vi "Update Function Variables.vi"(8 "error in (no error)":errorcluster, 10 "Variable Names":string[](array[string]), 11 "Structure Loop in":refnum<class "functionbase.lvclass">) -> (0 "error out":errorcluster, 3 "Structure Loop out":refnum<class "functionbase.lvclass">)   [LabVIEW 2019, in "LSL.lvlib" / "functionbase.lvclass"]
uses:
  functionbase.lvclass
  functionbase.lvclass/functionbase.ctl
  properties/Read Func Full String.vi
  properties/Read RT Variables.vi
  variables/RT Variables/RT Variables.lvclass
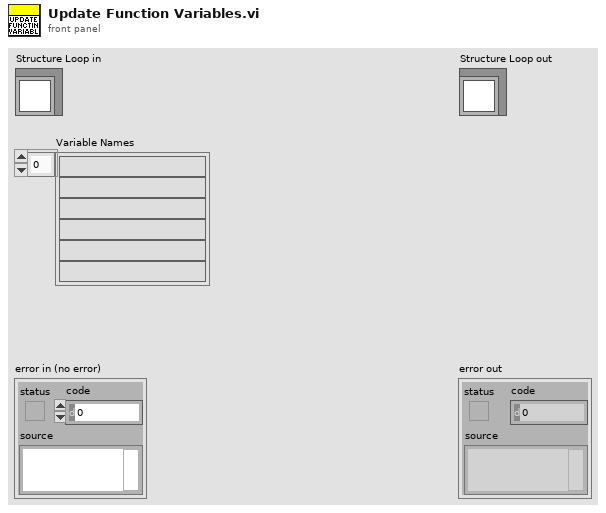
[diagram p1: front panel]
types:
  T1 = typedef "Datatype.ctl" = enum16{"Null", "Numeric", "String", "Bool", "Numeric 1D", "String 1D", "Bool 1D", "Numeric 2D", "String 2D", "Bool 2D", "Variant"}
  T2 = typedef "Valuetype.ctl" = enum16{"Value", "Variable", "Function"}
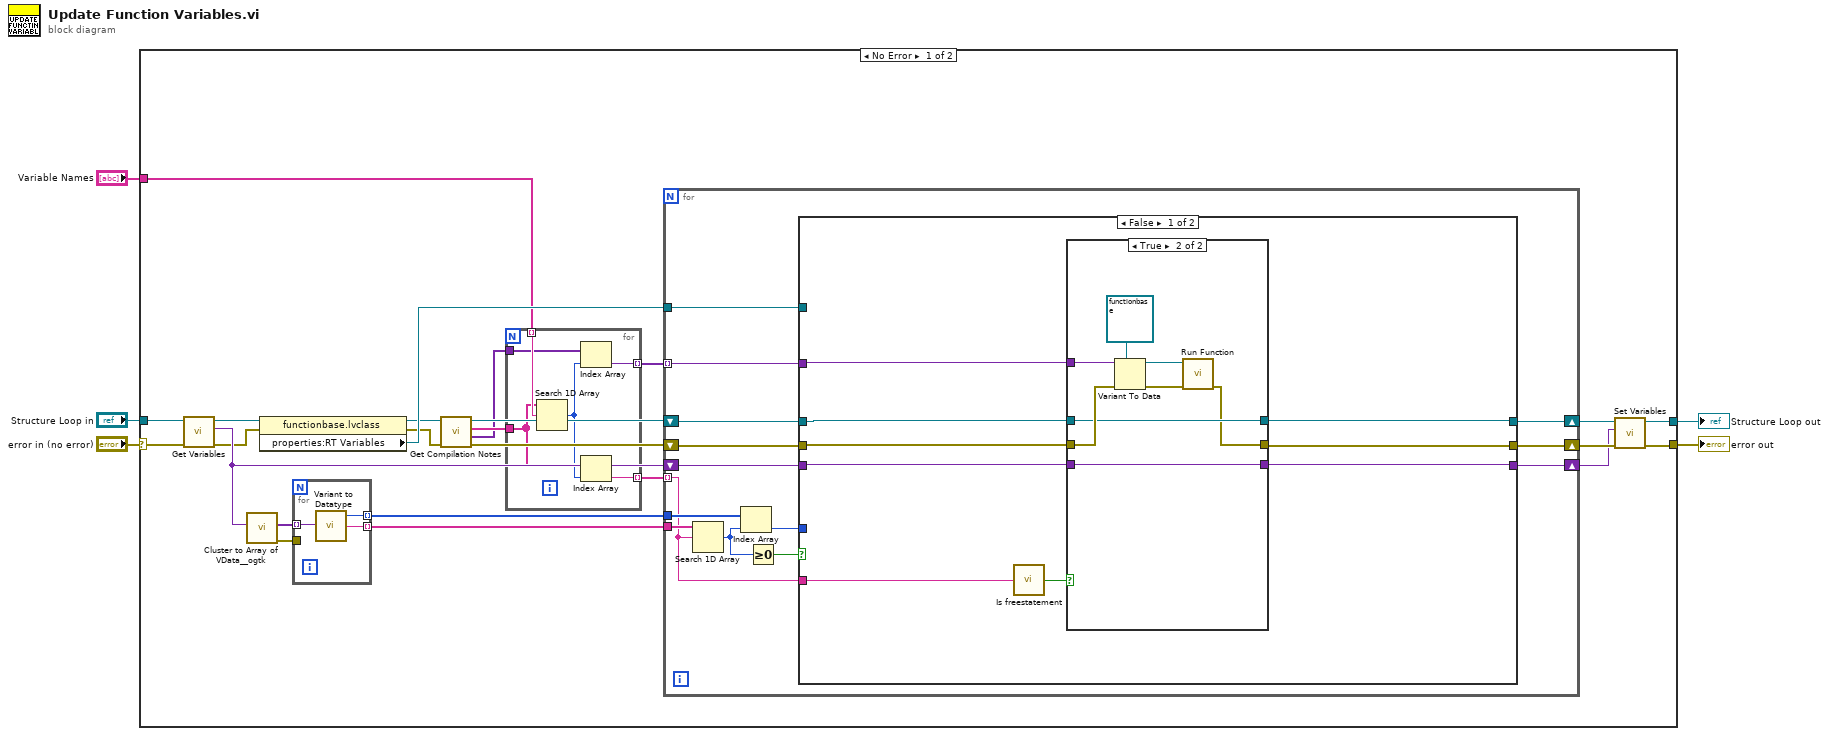
[diagram p0: block diagram]
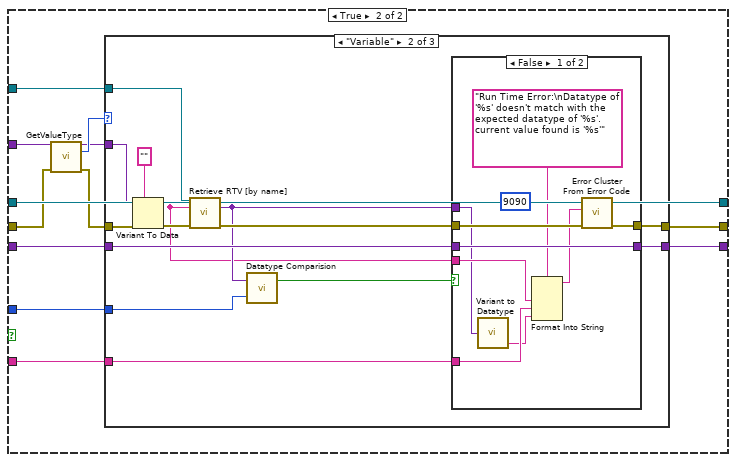
[diagram p3: hidden frame]
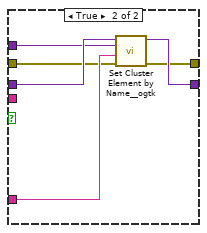
[diagram p5: hidden frame]
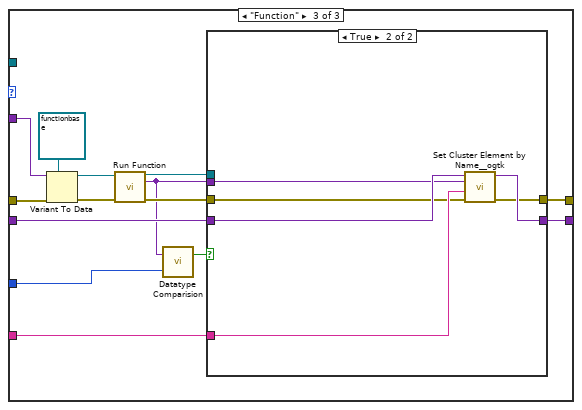
[diagram p6: hidden frame]
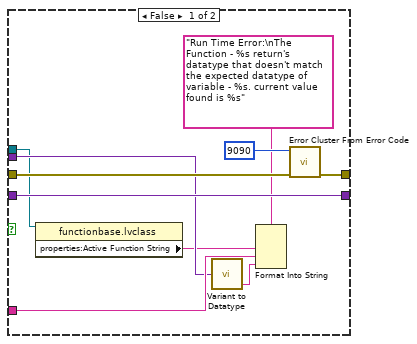
[diagram p7: hidden frame]
diagram:
  n1 = case shown="No Error" "error in (no error)" {
    selector: "error in (no error)" -> [w28 w148]
    tunnel: [w21 w148] -> w3
    tunnel: [w20 w147] -> w2
    tunnel: "Structure Loop in" -> [w27 w147]
    tunnel: "Variable Names" -> [w16 _]
    frame No Error {
      n2 = call-dynamic "Get Variables.vi"("error in (no error)"=w28, "functionbase in"=w27) -> ("error out"=w18:errorcluster, "Variables"=w25:variant, "functionbase out"=w19:refnum<class "functionbase.lvclass">)  [unwired: 7 in]
      n3 = call <userlib>:"Cluster to Array of VData__ogtk.vi"("Cluster"=w25) -> ("error out"=w26:errorcluster, "Array of VData"=w29:variant[])  [unwired: 9 in]
      n4 = property class="functionbase.lvclass"(reference=w19, error in=w18) -> (reference out=w15:refnum<class "functionbase.lvclass">, error out=w13:errorcluster, "properties:RT Variables"=w17:refnum<class "RT Variables.lvclass">)
      n5 = for {
        tunnel: w29 -> [w146] mode=indexing
        tunnel: [w145] -> w11 mode=indexing
        tunnel: [w144] -> w10 mode=indexing
        tunnel: w26 -> [_]
        n6 = call "Variant to Datatype.vi"("Variant"=w146) -> ("Name"=w144:string, "Datatype"=w145:T1)  [unwired: 2 in, 1 out]
      }
      n7 = call "Get Compilation Notes.vi"("error in (no error)"=w13, "functionbase in"=w15) -> ("error out"=w12:errorcluster, "note"=w8:variant[], "note Key"=w9:string[], "functionbase out"=w14:refnum<class "functionbase.lvclass">)  [unwired: 6 in]
      n8 = for {
        tunnel: w16 -> [w35] mode=indexing
        tunnel: w9 -> [w34]
        tunnel: w8 -> [w33]
        tunnel: [w31] -> w6 mode=indexing
        tunnel: [w30] -> w7 mode=indexing
        n9 = Search 1D Array(1D array=w34, element=w35) -> (index of element=w32:i32)  [unwired: 1 in]
        n10 = Index Array(array=w33, index=w32) -> (element=w30:variant)
        n11 = Index Array(array=w34, index=w32) -> (element=w31:string)
      }
      n12 = for {
        shift-right: [w46] -> w24
        shift-left: w14 -> [w42]
        tunnel: w10 -> [w41]
        shift-right: [w48] -> w22
        shift-left: w25 -> [w49]
        shift-right: [w47] -> w23
        shift-left: w12 -> [w43]
        tunnel: w11 -> [w40]
        tunnel: w17 -> [w45]
        tunnel: w7 -> [w44] mode=indexing
        tunnel: w6 -> [w38] mode=indexing
        n13 = Search 1D Array(1D array=w41, element=w38) -> (index of element=w37:i32)  [unwired: 1 in]
        n14 = Index Array(array=w40, index=w37) -> (element=w39:T1)
        n15 = Greater Or Equal To 0?(x=w37) -> (x >= 0?=w36:bool)
        n16 = case shown="False" w36 {
          tunnel: w49 -> [w57 w75]
          tunnel: [w56 w76] -> w48
          tunnel: w42 -> [w53 w81]
          tunnel: w43 -> [w54 w79]
          tunnel: w44 -> [w51 w80]
          tunnel: [w55 w74] -> w47
          tunnel: [w52 w81] -> w46
          tunnel: w39 -> [_ w72]
          tunnel: w38 -> [w50 w71]
          tunnel: w45 -> [_ w70]
          frame False {
            n17 = call "Is freestatement.vi"("Variable Name"=w50) -> ("freestatement?"=w58:bool)
            n18 = case shown="True" w58 {
              tunnel: w54 -> [w61 w66]
              tunnel: [w61 w63] -> w55
              tunnel: [w60 w65] -> w52
              tunnel: w53 -> [w60 w65]
              tunnel: [w59 w62] -> w56
              tunnel: w57 -> [w59 w62]
              tunnel: w51 -> [_ w64]
              frame False {
              }
              frame True {
                n19 = Variant To Data(error in=w66, type=refnum<class "functionbase.lvclass"> refnum ("functionbase.lvclass"), Variant=w64) -> (data=w67:refnum<class "functionbase.lvclass">, error out=w68:errorcluster)
                n20 = call-dynamic "Run Function.vi"("functionbase in"=w67, "error in (no error)"=w68) -> ("error out"=w63:errorcluster)  [unwired: 11 in, 2 out]
              }
            }
          }
          frame True {
            n21 = call "GetValueType.vi"("variant"=w80, "error in"=w79) -> ("variant out"=w77:variant, "Value Type"=w78:T2, "error out"=w73:errorcluster)  [unwired: 11 in]
            n22 = case shown="\"Variable\"" w78 {
              tunnel: w77 -> [_ w96 w126]
              tunnel: [w83 w92 w122] -> w76
              tunnel: w75 -> [w83 w93 w123]
              tunnel: [w82 w91 w119] -> w74
              tunnel: w73 -> [w82 w97 w127]
              tunnel: w72 -> [_ w88 w117]
              tunnel: w71 -> [_ w89 w121]
              tunnel: w70 -> [_ w86 _]
              frame "Value", Default {
              }
              frame "Variable" {
                n23 = Variant To Data(error in=w97, type="", Variant=w96) -> (data=w84:string, error out=w94:errorcluster)
                n24 = call-dynamic "Retrieve RTV [by name].vi"("RT Variables in"=w86, "RTV name"=w84, "error in (no error)"=w94) -> ("Data"=w85:variant, "error out"=w90:errorcluster)  [unwired: 8 in, 3 out]
                n25 = call "Datatype Comparision.vi"("Required Datatype"=w88, "Data"=w85) -> ("Equal?"=w87:bool)  [unwired: 1 out]
                n26 = case shown="False" w87 {
                  tunnel: w93 -> [w107 w113]
                  tunnel: [w107 w112] -> w92
                  tunnel: w85 -> [w99 w111]
                  tunnel: w89 -> [w100 w110]
                  tunnel: w90 -> [w106 w109]
                  tunnel: [w105 w108] -> w91
                  tunnel: w84 -> [w101 _]
                  frame False {
                    n27 = call "Variant to Datatype.vi"("Variant"=w99) -> ("Value"=w98:string)  [unwired: 2 in, 2 out]
                    n28 = Format Into String(format string="Run Time Error:\nDatatype of '%s' doesn't match with the expected datatype of '%s'. current value found is '%s'" ("error message (\"\")"), w101, w100, w98) -> (resulting string=w102:string)  [unwired: 2 in, 1 out]
                    n29 = call <vilib>:"Error Cluster From Error Code.vi"("error in (no error)"=w106, "error message (\"\")"=w102, "error code (0)"=9090) -> ("error out"=w105:errorcluster)  [unwired: 6 in]
                  }
                  frame True {
                    n30 = call <userlib>:"Set Cluster Element by Name__ogtk.vi"("error in (no error)"=w109, "Element Name (\"\": New Element Data Name)"=w110, "New Element Value"=w111, "Cluster"=w113) -> ("error out"=w108:errorcluster, "VCluster out"=w112:variant)  [unwired: 5 in, 1 out]
                  }
                }
              }
              frame "Function" {
                n31 = Variant To Data(error in=w127, type=refnum<class "functionbase.lvclass"> refnum ("functionbase.lvclass"), Variant=w126) -> (data=w115:refnum<class "functionbase.lvclass">, error out=w124:errorcluster)
                n32 = call-dynamic "Run Function.vi"("functionbase in"=w115, "error in (no error)"=w124) -> ("functionbase out"=w114:refnum<class "functionbase.lvclass">, "Return"=w118:variant, "error out"=w120:errorcluster)  [unwired: 11 in]
                n33 = call "Datatype Comparision.vi"("Required Datatype"=w117, "Data"=w118) -> ("Equal?"=w116:bool)  [unwired: 1 out]
                n34 = case shown="True" w116 {
                  tunnel: w123 -> [w137 w143]
                  tunnel: [w137 w142] -> w122
                  tunnel: w118 -> [w130 w141]
                  tunnel: w121 -> [w131 w140]
                  tunnel: w120 -> [w136 w139]
                  tunnel: [w135 w138] -> w119
                  tunnel: w114 -> [w129 _]
                  frame False {
                    n35 = property class="functionbase.lvclass"(reference=w129) -> ("properties:Active Function String"=w128:string)  [unwired: 1 in, 2 out]
                    n36 = call "Variant to Datatype.vi"("Variant"=w130) -> ("Value"=w133:string)  [unwired: 2 in, 2 out]
                    n37 = Format Into String(format string="Run Time Error:\nThe Function - %s return's datatype that doesn't match the expected datatype of variable - %s. current value found is %s" ("error message (\"\")"), w128, w131, w133) -> ()  [unwired: 2 in, 2 out]
                    n38 = call <vilib>:"Error Cluster From Error Code.vi"("error in (no error)"=w136, "error code (0)"=9090) -> ("error out"=w135:errorcluster)  [unwired: 7 in]
                  }
                  frame True {
                    n39 = call <userlib>:"Set Cluster Element by Name__ogtk.vi"("error in (no error)"=w139, "Element Name (\"\": New Element Data Name)"=w140, "New Element Value"=w141, "Cluster"=w143) -> ("error out"=w138:errorcluster, "VCluster out"=w142:variant)  [unwired: 5 in, 1 out]
                  }
                }
              }
            }
          }
        }
      }
      n40 = call-dynamic "Set Variables.vi"("error in (no error)"=w23, "Variables"=w22, "functionbase in"=w24) -> ("error out"=w21:errorcluster, "functionbase out"=w20:refnum<class "functionbase.lvclass">)  [unwired: 7 in]
    }
    frame Error {
    }
  }
  "error out" <- w3
  "Structure Loop out" <- w2
